vi "MercuryRemoteTest.vi"() -> ()   [LabVIEW 2013]
panel:
  out "Mercury Status":string
  in  "stop":bool
  out "Mercury Targets 2":T1
  out "Mercury actions":T2
  in  "Mercury Targets":T1
  in  "mercury actions":T2
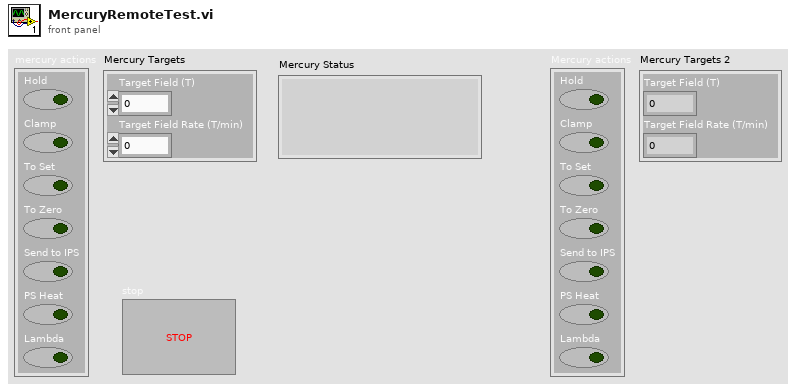
[diagram p1: front panel]
types:
  T1 = cluster{"Target Field (T)":dbl, "Target Field Rate (T/min)":dbl}
  T2 = cluster{"Hold":bool, "Clamp":bool, "To Set":bool, "To Zero":bool, "Send to IPS":bool, "PS Heat":bool, "Lambda":bool}
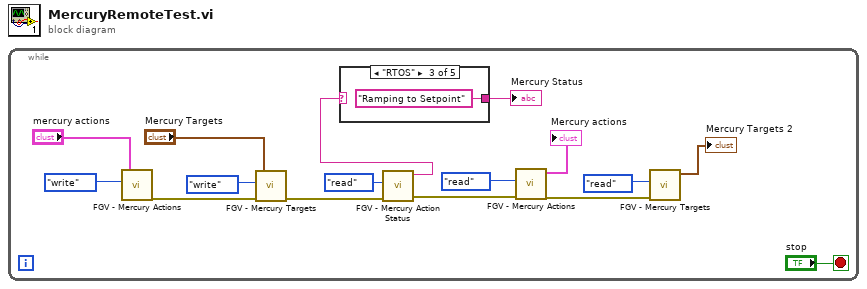
[diagram p0: block diagram]
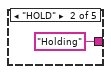
[diagram p3: hidden frame]
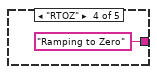
[diagram p4: hidden frame]
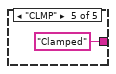
[diagram p5: hidden frame]
diagram:
  n1 = while {
    stop <- "stop" stop-if-true
    n2 = call "FGV - Mercury Actions.vi"("Function"=enum16{"write", "read"}."write", "mercury actions"="mercury actions") -> ("error out"=w11:errorcluster)  [unwired: 4 in, 1 out]
    n3 = call "FGV - Mercury Targets.vi"("error in"=w11, "Function"=enum16{"write", "read"}."write", "Mercury Targets"="Mercury Targets") -> ("error out"=w10:errorcluster)  [unwired: 3 in, 1 out]
    n4 = call "FGV - Mercury Action Status.vi"("error in"=w10, "Function"=enum16{"write", "read"}."read") -> ("error out"=w6:errorcluster, "Mercury Status"=w2:string)  [unwired: 4 in]
    n5 = case shown="\"RTOS\"" w2 {
      selector: w2 -> [w17 _ _ _ _]
      tunnel: [w17 "Holding" "Ramping to Setpoint" "Ramping to Zero" "Clamped"] -> w1
      frame Default {
      }
      frame "HOLD" {
      }
      frame "RTOS" {
      }
      frame "RTOZ" {
      }
      frame "CLMP" {
      }
    }
    "Mercury Status" <- w1
    n6 = call "FGV - Mercury Actions.vi"("error in"=w6, "Function"=enum16{"write", "read"}."read") -> ("error out"=w9:errorcluster, "Mercury actions"=→"Mercury actions":T2)  [unwired: 4 in]
    n7 = call "FGV - Mercury Targets.vi"("error in"=w9, "Function"=enum16{"write", "read"}."read") -> ("Mercury Targets"=→"Mercury Targets 2":T1)  [unwired: 4 in, 1 out]
  }
